vi "Delete null array.vi"(11 "Array In":dbl[][](array[numeric])=[[0.0, 2.0, 0.0]]) -> (0 "Rows and columns deleted":dbl[][](array[numeric])=[[2.0]], 3 "Only rows deleted":dbl[][](array[numeric])=[[2.0]])   [LabVIEW 2020]
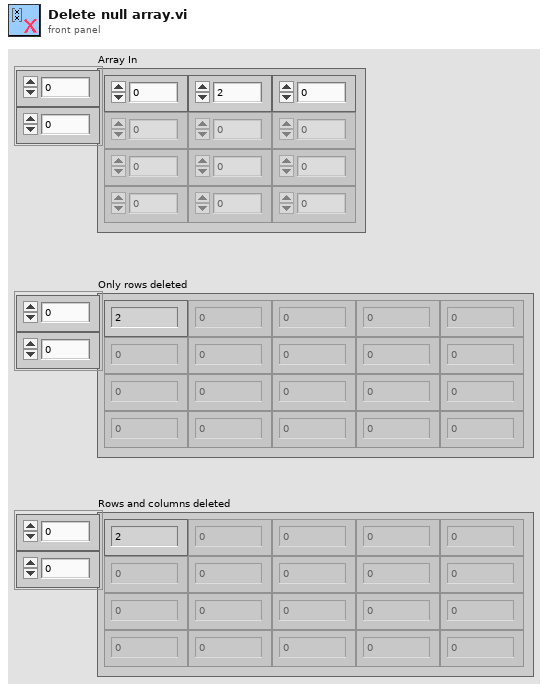
[diagram p1: front panel]
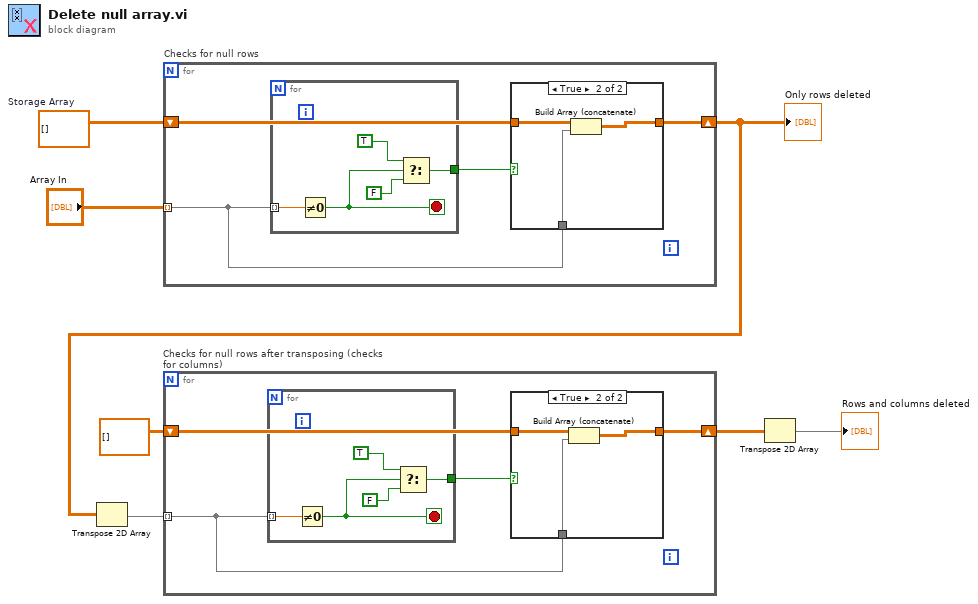
[diagram p0: block diagram]
diagram:
  w6 = dbl[][] []  # Storage Array
  n1 = for "Checks for null rows" {
    tunnel: "Array In" -> [w10] mode=indexing
    shift-right: [w8] -> w4
    shift-left: w6 -> [w9]
    n2 = for {
      tunnel: w10 -> [w16] mode=indexing
      tunnel: [w14] -> w11
      stop <- w15 stop-if-true
      n3 = Not Equal To 0?(x=w16) -> (x != 0?=w15:bool)
      n4 = Select(t=TRUE, s=w15, f=FALSE) -> (s? t:f=w14:bool)
    }
    n5 = case "If \"F\" then \nadd row to results." shown="True" w11 {
      tunnel: [w17 w19] -> w8
      tunnel: w10 -> [_ w18]
      tunnel: w9 -> [w17 w20]
      frame False {
      }
      frame True {
        n6 = Build Array (concatenate)(w20, w18) -> (w19:dbl[][])
      }
    }
  }
  "Only rows deleted" <- w4
  n7 = Transpose 2D Array(2D array=w4) -> (transposed array=w2:dbl[][])
  n8 = for "Checks for null rows after transposing (checks for columns)" {
    tunnel: w2 -> [w23] mode=indexing
    shift-right: [w21] -> w3
    shift-left: dbl[][] [] -> [w22]
    n9 = for {
      tunnel: w23 -> [w29] mode=indexing
      tunnel: [w27] -> w24
      stop <- w28 stop-if-true
      n10 = Not Equal To 0?(x=w29) -> (x != 0?=w28:bool)
      n11 = Select(t=TRUE, s=w28, f=FALSE) -> (s? t:f=w27:bool)
    }
    n12 = case "If \"F\" then \nadd row to results." shown="True" w24 {
      tunnel: [w30 w32] -> w21
      tunnel: w23 -> [_ w31]
      tunnel: w22 -> [w30 w33]
      frame False {
      }
      frame True {
        n13 = Build Array (concatenate)(w33, w31) -> (w32:dbl[][])
      }
    }
  }
  n14 = Transpose 2D Array(2D array=w3) -> (transposed array=→"Rows and columns deleted":dbl[][])
